vi "Check shutter.vi"(0 "SHUTTER":string(combo), 1 "MONOCHOMATOR":refnum<visa-resource-name>) -> (2 "SHUTTER STATUS":string="SHUTTER O")   [LabVIEW 2024]
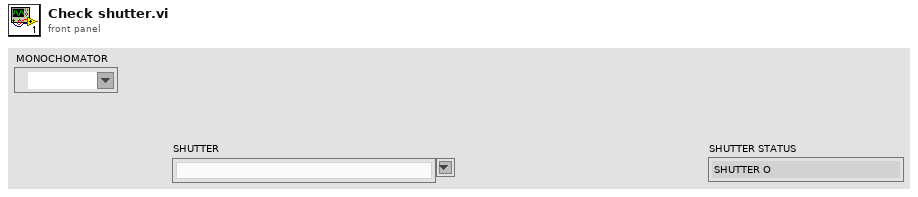
[diagram p1: front panel]
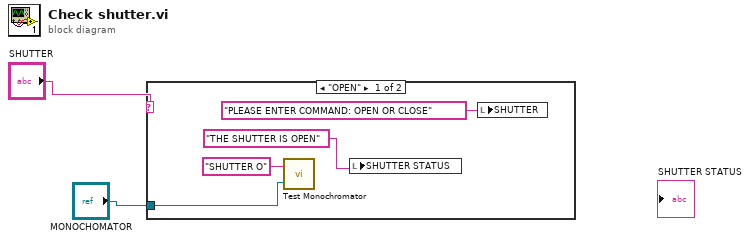
[diagram p0: block diagram]
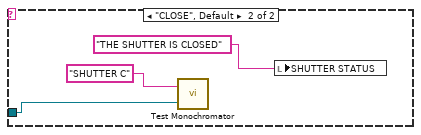
[diagram p2: hidden frame]
diagram:
  n1 = case shown="\"OPEN\"" "SHUTTER" {
    tunnel: "MONOCHOMATOR" -> [w3 w7]
    frame "OPEN" {
      n2 = call "Test Monochromator.vi"("MONOCHOMATOR"=w3, "Command"="SHUTTER O") -> ()  [unwired: 1 in, 1 out]
      n3 = local write "SHUTTER STATUS"("THE SHUTTER IS OPEN" ("String")) -> ()
      n4 = local write "SHUTTER"("PLEASE ENTER COMMAND: OPEN OR CLOSE") -> ()
    }
    frame "CLOSE", Default {
      n5 = call "Test Monochromator.vi"("MONOCHOMATOR"=w7, "Command"="SHUTTER C") -> ()  [unwired: 1 in, 1 out]
      n6 = local write "SHUTTER STATUS"("THE SHUTTER IS CLOSED" ("String")) -> ()
    }
  }
